vi "Configure Event Data.vi"(0 "VISA resource name":refnum<visa-resource-name>, 1 "Data Length (3: 1h)":u16(ring)=3 items=["10min", "20min", "30min", "1h", "2h", "3h", "4h", "6h", "8h", "12h", "1day", "2day", "3day", "5day", "7day", "14day", "31day", "2min", "5min"], 2 "Pre-Trigger (0: 0%)":u16(ring) items=["0%", "5%", "25%", "50%", "75%", "95%", "100%"], 3 "Trigger Source Operation (On)":bool=TRUE, 5 "Measurement Group (1)":i32=1 min=1 max=2, 7 "Recording Interval (3: 1s)":u16(ring)=3 items=["100ms", "200ms", "500ms", "1s", "2s", "5s", "10s", "15s", "20s", "30s", "1min", "2min", "5min", "10min", "15min", "20min", "30min", "1ms", "2ms", "5ms", "10ms", "20ms", "50ms"], 9 "Recording Mode (0: Free)":u16(ring) items=["Free", "Single", "Repeat"], 11 "error in (no error)":errorcluster) -> (4 "VISA resource name out":refnum<visa-resource-name>, 6 "Measurement Group":i32, 15 "error out":errorcluster)   [LabVIEW 2020, in "Yokogawa GX Series.lvlib"]
doc: "Sets the event data recording mode.\n\nCommand: SEventData"
uses:
  <instrlib>/Yokogawa GX Series/Yokogawa GX Series.lvlib
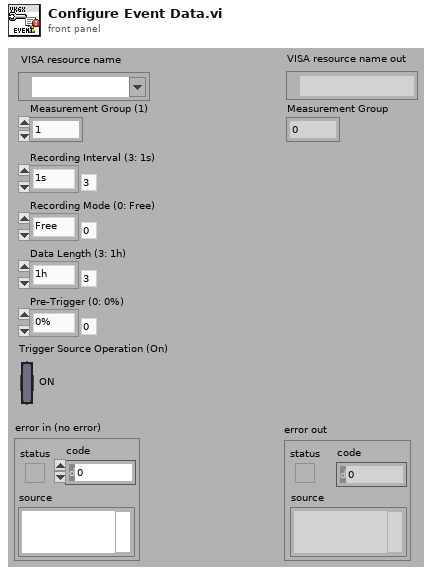
[diagram p1: front panel]
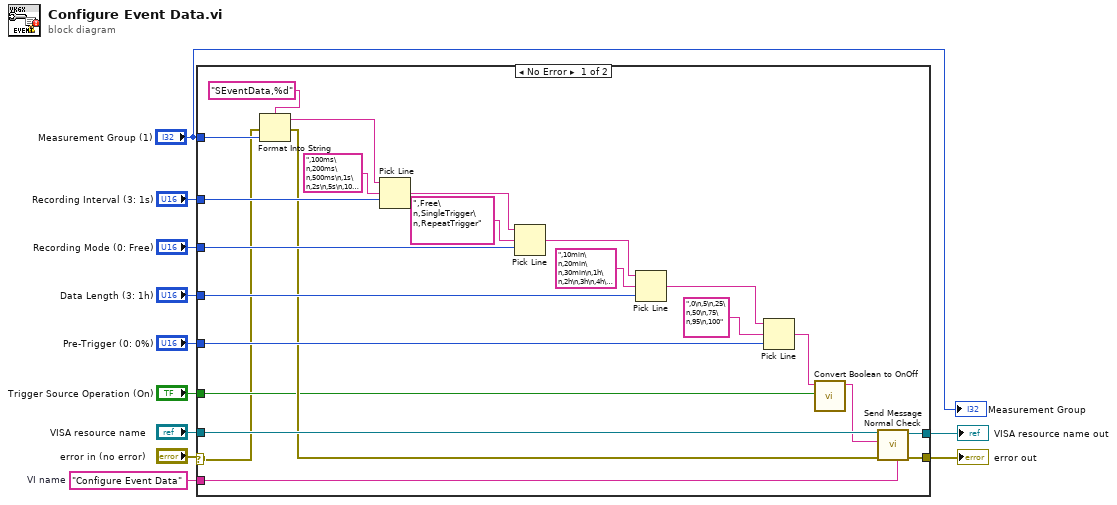
[diagram p0: block diagram]
diagram:
  w11 = "Configure Event Data"  # VI name
  n1 = case shown="No Error" "error in (no error)" {
    selector: "error in (no error)" -> [w12 w35]
    tunnel: w11 -> [w34 _]
    tunnel: [w33 w36] -> w10
    tunnel: [w32 w35] -> w9
    tunnel: "VISA resource name" -> [w31 w36]
    tunnel: "Recording Interval (3: 1s)" -> [w29 _]
    tunnel: "Recording Mode (0: Free)" -> [w26 _]
    tunnel: "Data Length (3: 1h)" -> [w23 _]
    tunnel: "Pre-Trigger (0: 0%)" -> [w20 _]
    tunnel: "Measurement Group (1)" -> [w16 _]
    tunnel: "Trigger Source Operation (On)" -> [w15 _]
    frame No Error {
      n2 = Format Into String(format string="SEventData,%d", error in=w12, w16) -> (resulting string=w17:string, error out=w18:errorcluster)  [unwired: 1 in]
      n3 = Pick Line(string ("")=w17, multi-line string=",100ms\n,200ms\n,500ms\n,1s\n,2s\n,5s\n,10s\n,15s\n,20s\n,30s\n,1min\n,2min\n,5min\n,10min\n,15min\n,20min\n,30min\n,1ms\n,2ms\n,5ms\n,10ms\n,20ms\n,50ms", line index=w29) -> (output string=w28:string)
      n4 = Pick Line(string ("")=w28, multi-line string=",Free\n,SingleTrigger\n,RepeatTrigger", line index=w26) -> (output string=w25:string)
      n5 = Pick Line(string ("")=w25, multi-line string=",10min\n,20min\n,30min\n,1h\n,2h\n,3h\n,4h\n,6h\n,8h\n,12h\n,1day\n,2day\n,3day\n,5day\n,7day\n,14day\n,31day\n,2min\n,5min", line index=w23) -> (output string=w22:string)
      n6 = Pick Line(string ("")=w22, multi-line string=",0\n,5\n,25\n,50\n,75\n,95\n,100", line index=w20) -> (output string=w14:string)
      n7 = call <instrlib>:"Convert Boolean to OnOff.vi"("On/Off"=w15, "Initial String (\"\")"=w14) -> ("Resulting String"=w13:string)  [unwired: 9 in]
      n8 = call <instrlib>:"Send Message Normal Check.vi"("Source (\"\")"=w34, "error in (no error)"=w18, "Send Message (\"\")"=w13, "VISA resource name"=w31) -> ("error out"=w32:errorcluster, "VISA resource name out"=w33:refnum<visa-resource-name>)  [unwired: 2 in, 4 out]
    }
    frame Error {
    }
  }
  "error out" <- w9
  "VISA resource name out" <- w10
  "Measurement Group" <- "Measurement Group (1)"
